vi "Global 1.vi"() -> ()   [LabVIEW 2019]
panel:
  out "unser x wert":dbl
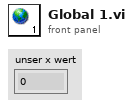
[diagram p1: front panel]
diagram:
